vi "Decode.vi"(8 "error in (no error)":errorcluster, 11 "JSON in":string) -> (0 "error out":errorcluster, 3 "Variant out":variant)   [LabVIEW 2019, in "JSON.lvlib"]
doc: "Decodes the JSON string to a LabVIEW Variant where JSON objects are represented as LabVIEW Clusters.\n\nEmpty JSON objects (\"{}\") are represented as a Cluster with an U16 Enum <b>\"empty\"</b> placeholder. \nNull JSON values (\"NULL\") are represented as a U8 Enum <b>\"null\"</b> placeholder. \nElements in JSON arrays are represented as Variant values.\nTimestamps are JSON strings formatted as defined in RFC-3339 (\"yyyy-mm-ddThh:mm:ss.uuuuuu\").\n\nCreated by: Ryan Pacini"
uses:
  JSON.lvlib
  <vilib>/regexp/Match Regular Expression.xnode
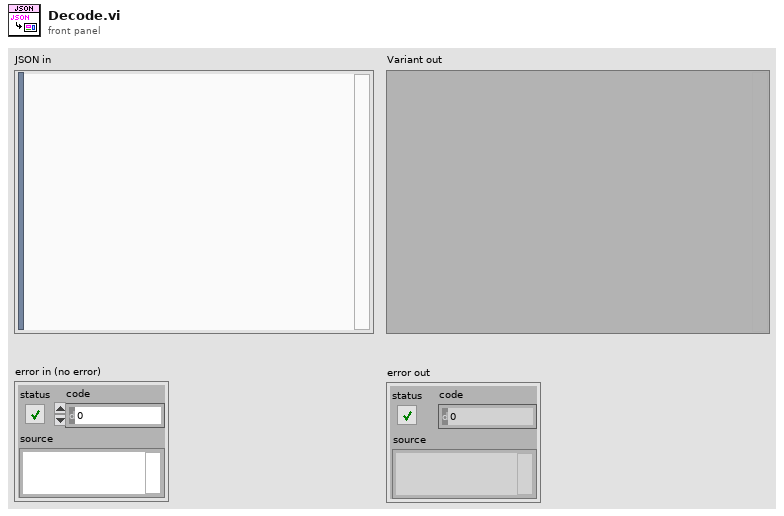
[diagram p1: front panel]
types:
  T1 = cluster{"k":string, "t":enum8{"root", "array", "object"}, "v":variant[]}[]
  T2 = cluster{"k":string, "t":enum8{"root", "array", "object"}, "v":variant[]}
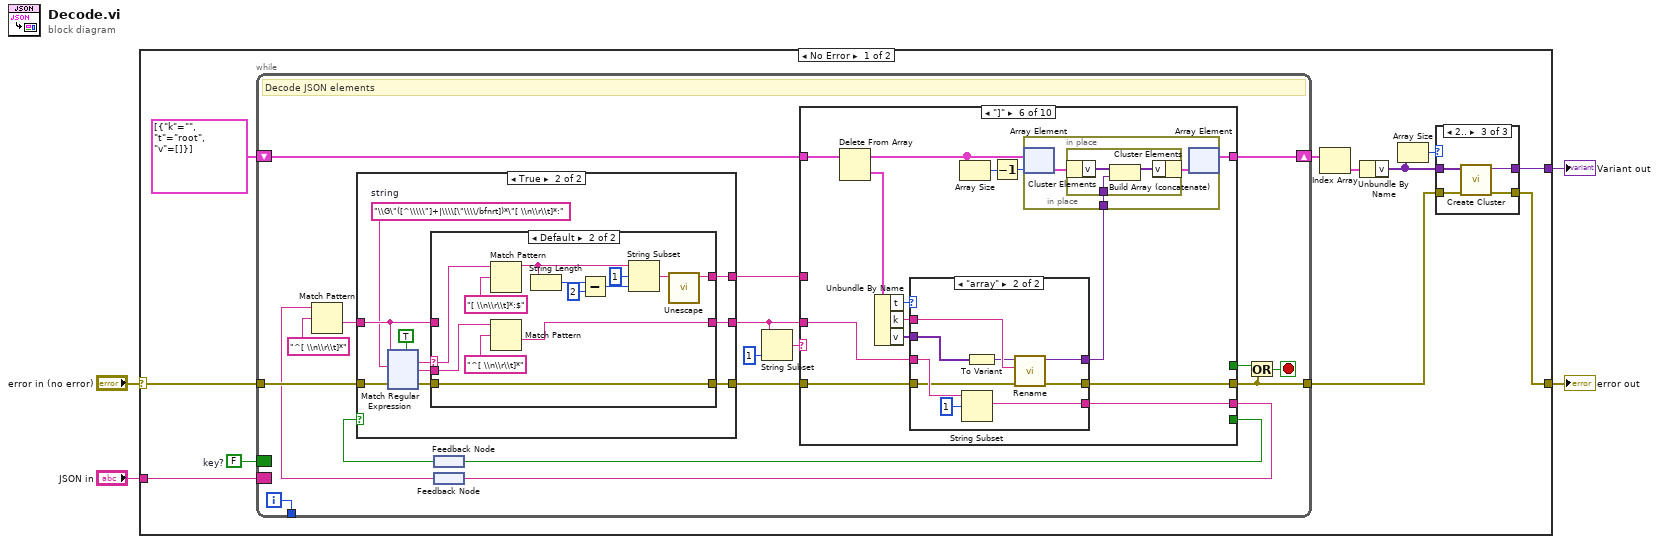
[diagram p0: block diagram]
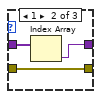
[diagram p3: hidden frame]
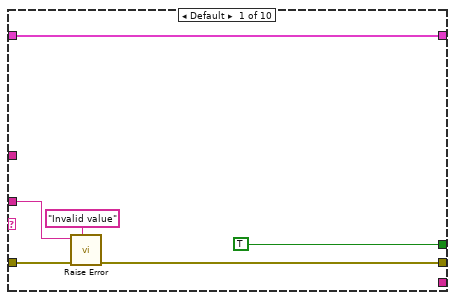
[diagram p4: hidden frame]
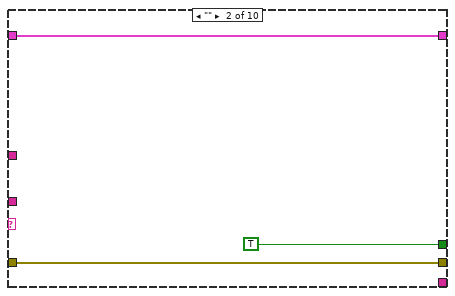
[diagram p5: hidden frame]
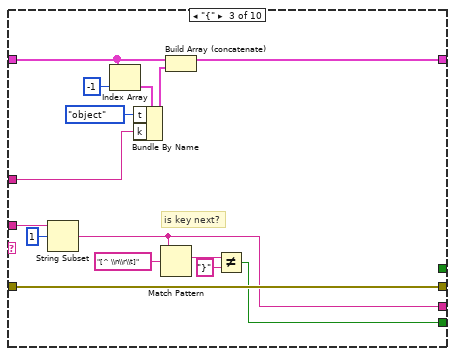
[diagram p6: hidden frame]
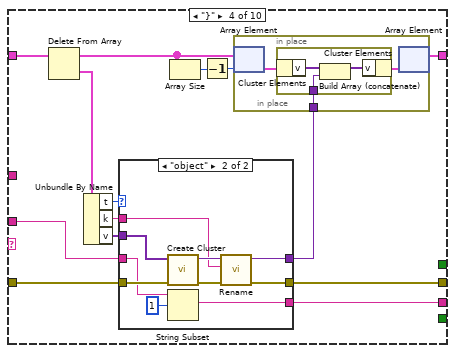
[diagram p7: hidden frame]
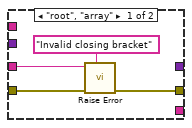
[diagram p8: hidden frame]
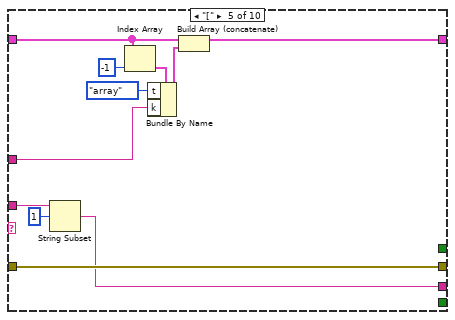
[diagram p9: hidden frame]
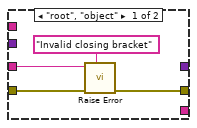
[diagram p10: hidden frame]
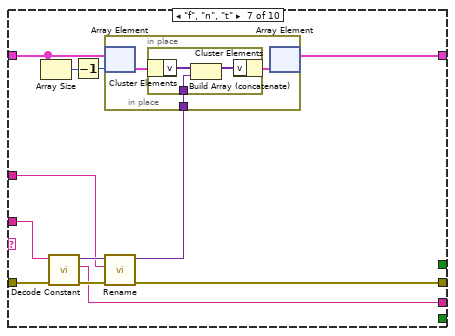
[diagram p11: hidden frame]
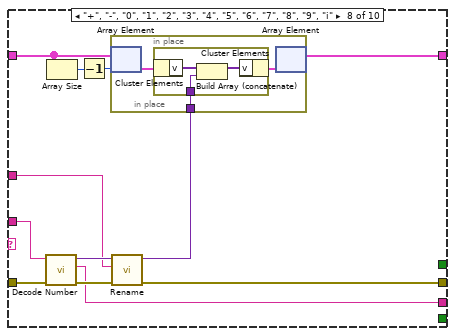
[diagram p12: hidden frame]
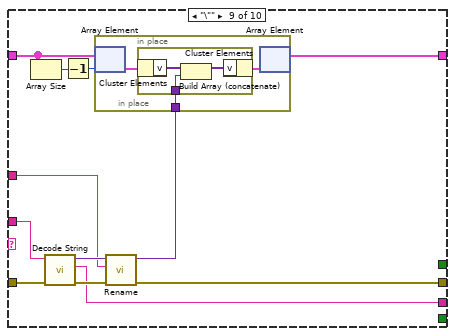
[diagram p13: hidden frame]
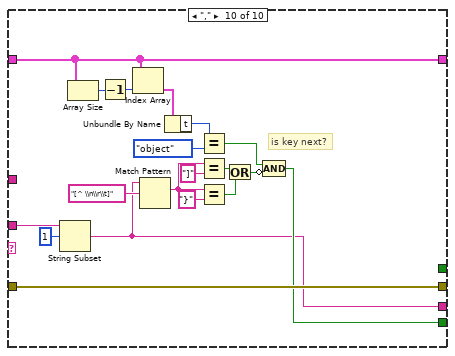
[diagram p14: hidden frame]
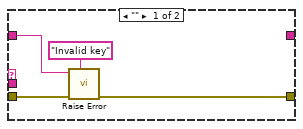
[diagram p16: hidden frame]
diagram:
  n1 = case shown="No Error" "error in (no error)" {
    selector: "error in (no error)" -> [w15 w360]
    tunnel: "JSON in" -> [w13 _]
    tunnel: [w5 w360] -> w2
    tunnel: [w8 _] -> w1
    frame No Error {
      w12 = FALSE  # key?
      n2 = while {
        tunnel: w15 -> [w41]
        shift-right: [w38] -> w11
        shift-left: T1 [{"k"="", "t"=enum."root", "v"=[]}] ("e") -> [w39]
        tunnel: [w36] -> w6
        border: w13 -> [_]
        border: w12 -> [_]
        tunnel: [w24] -> _
        i -> [w24]
        stop <- w34 stop-if-true
        # "Decode JSON elements"
        n3 = feedback #1() -> (w28:bool)
        n4 = feedback #2() -> (w32:string)
        n5 = Match Pattern(string=w32, regular expression="^[ \\n\\r\\t]*") -> (after substring=w31:string)  [unwired: 1 in, 3 out]
        n6 = case shown="True" w28 {
          tunnel: w41 -> [w218 w223]
          tunnel: w31 -> [w217 w225]
          tunnel: [w218 w226] -> w40
          tunnel: [_ w221] -> w37
          tunnel: [w217 w219] -> w27
          frame False {
          }
          frame True {
            w224 = "\\G\"([^\\\\\"]+|\\\\[\"\\\\/bfnrt])*\"[ \\n\\r\\t]*:"  # string
            n7 = xnode "Match Regular Expression"("input string"=w225, "regular expression"=w224, "error in"=w223, "multiline? (F)"=TRUE) -> ("whole match"=w227:string, "after match"=w220:string, "error out"=w222:errorcluster)  [unwired: 2 in, 2 out]
            n8 = case shown="Default" w227 {
              selector: w227 -> [_ w243]
              tunnel: w225 -> [w229 _]
              tunnel: [w231 w245] -> w226
              tunnel: w222 -> [w232 w245]
              tunnel: [_ w240] -> w221
              tunnel: w220 -> [_ w234]
              tunnel: [_ w233] -> w219
              frame "" {
                n9 = call "Raise Error.vi"("message"="Invalid key", "error in (no error)"=w232, "json"=w229) -> ("error out"=w231:errorcluster)  [unwired: 8 in]
              }
              frame Default {
                n10 = Match Pattern(string=w243, regular expression="[ \\n\\r\\t]*:$") -> (before substring=w239:string)  [unwired: 1 in, 3 out]
                n11 = Match Pattern(string=w234, regular expression="^[ \\n\\r\\t]*") -> (after substring=w233:string)  [unwired: 1 in, 3 out]
                n12 = String Length(string=w239) -> (length=w237:i32)
                n13 = Subtract(x=w237, y=2 ("x")) -> (x-y=w236:i32)
                n14 = String Subset(string=w239, offset (0)=1, length (rest)=w236) -> (substring=w241:string)
                n15 = call "Unescape.vi"("escaped string"=w241) -> ("string out"=w240:string)  [unwired: 9 in, 1 out]
              }
            }
          }
        }
        n16 = String Subset(string=w27, length (rest)=1 ("length (rest)")) -> (substring=w29:string)  [unwired: 1 in]
        n17 = case shown="\"]\"" w29 {
          tunnel: w40 -> [w44 w48 w65 w73 w110 w118 w155 w173 w191 w216]
          tunnel: [w43 w48 w65 w71 w110 w116 w148 w166 w184 w216] -> w36
          tunnel: w39 -> [w47 w50 w57 w79 w106 w124 w152 w169 w187 w206]
          tunnel: [w47 w50 w64 w74 w109 w119 w153 w168 w186 w206] -> w38
          tunnel: w37 -> [_ _ w60 _ w107 _ w146 w163 w181 _]
          tunnel: [_ _ w61 _ _ _ _ _ _ w207] -> w26
          tunnel: w27 -> [w42 _ w53 w68 w102 w112 w154 w172 w190 w201]
          tunnel: [TRUE TRUE _ _ _ _ _ _ _ _] -> w35
          tunnel: [_ _ w52 w67 w101 w111 w144 w164 w182 w199] -> w25
          frame Default {
            n18 = call "Raise Error.vi"("message"="Invalid value" ("source"), "error in (no error)"=w44, "json"=w42) -> ("error out"=w43:errorcluster)  [unwired: 8 in]
          }
          frame "" {
          }
          frame "{" {
            # "is key next?"
            n19 = String Subset(string=w53, offset (0)=1) -> (substring=w52:string)  [unwired: 1 in]
            n20 = Index Array(array=w57, index=-1) -> (element=w55:T2)
            n21 = Bundle By Name(cluster=w55, "t"=enum8{"root", "array", "object"}."object", "k"=w60) -> (w63:T2)
            n22 = Match Pattern(string=w52, regular expression="[^ \\n\\r\\t]") -> (match substring=w58:string)  [unwired: 1 in, 3 out]
            n23 = Build Array (concatenate)(w57, w63) -> (w64:T1)
            n24 = Not Equal?(x=w58, y="}") -> (x != y?=w61:bool)
          }
          frame "}" {
            n25 = Delete From Array(array=w79) -> (deleted portion=w78:T2, array with subset deleted=w75:T1)  [unwired: 2 in]
            n26 = Unbundle By Name(w78) -> ("t"=w69:enum8{"root", "array", "object"}, "k"=w70:string, "v"=w72:variant[])
            n27 = case shown="\"object\"" w69 {
              tunnel: w73 -> [w82 w93]
              tunnel: w72 -> [_ w84]
              tunnel: [w81 w91] -> w71
              tunnel: w70 -> [_ w89]
              tunnel: [_ w88] -> w66
              tunnel: w68 -> [w80 w85]
              tunnel: [_ w86] -> w67
              frame "root", "array" {
                n28 = call "Raise Error.vi"("message"="Invalid closing bracket", "error in (no error)"=w82, "json"=w80) -> ("error out"=w81:errorcluster)  [unwired: 8 in]
              }
              frame "object" {
                n29 = call "Create Cluster.vi"("error in (no error)"=w93, "elements"=w84) -> ("error out"=w92:errorcluster, "cluster"=w90:variant)  [unwired: 8 in]
                n30 = String Subset(string=w85, offset (0)=1) -> (substring=w86:string)  [unwired: 1 in]
                n31 = call "Rename.vi"("error in (no error)"=w92, "name"=w89, "variant in"=w90) -> ("error out"=w91:errorcluster, "variant out"=w88:variant)  [unwired: 7 in]
              }
            }
            n32 = Array Size(array=w75) -> (size(s)=w77:i32)
            n33 = Decrement(x=w77) -> (x-1=w76:i32)
            n34 = in-place {
              in-place-border: w66 -> [w95]
              n35 = in-place-array #3(w75, w76) -> (w96:T2)
              n36 = in-place {
                in-place-border: w95 -> [w97]
                n37 = in-place-cluster #4(w96) -> ("v"=w99:variant[])
                n38 = Build Array (concatenate)(w99, w97) -> (w98:variant[])
                n39 = in-place-cluster #4("v"=w98) -> (w94:T2)
              }
              n40 = in-place-array #3(w94) -> (w74:T1)  [unwired: 1 out]
            }
          }
          frame "[" {
            n41 = String Subset(string=w102, offset (0)=1) -> (substring=w101:string)  [unwired: 1 in]
            n42 = Index Array(array=w106, index=-1) -> (element=w105:T2)
            n43 = Bundle By Name(cluster=w105, "t"=enum8{"root", "array", "object"}."array", "k"=w107) -> (w108:T2)
            n44 = Build Array (concatenate)(w106, w108) -> (w109:T1)
          }
          frame "]" {
            n45 = Delete From Array(array=w124) -> (deleted portion=w123:T2, array with subset deleted=w120:T1)  [unwired: 2 in]
            n46 = Unbundle By Name(w123) -> ("t"=w113:enum8{"root", "array", "object"}, "k"=w115:string, "v"=w117:variant[])
            n47 = case shown="\"array\"" w113 {
              tunnel: w118 -> [w127 w129]
              tunnel: w117 -> [_ w131]
              tunnel: [w126 w137] -> w116
              tunnel: w115 -> [_ w136]
              tunnel: [_ w135] -> w114
              tunnel: w112 -> [w125 w133]
              tunnel: [_ w132] -> w111
              frame "root", "object" {
                n48 = call "Raise Error.vi"("message"="Invalid closing bracket", "error in (no error)"=w127, "json"=w125) -> ("error out"=w126:errorcluster)  [unwired: 8 in]
              }
              frame "array" {
                n49 = String Subset(string=w133, offset (0)=1) -> (substring=w132:string)  [unwired: 1 in]
                n50 = To Variant(anything=w131) -> (Variant=w130:variant)
                n51 = call "Rename.vi"("error in (no error)"=w129, "name"=w136, "variant in"=w130) -> ("error out"=w137:errorcluster, "variant out"=w135:variant)  [unwired: 7 in]
              }
            }
            n52 = Array Size(array=w120) -> (size(s)=w122:i32)
            n53 = Decrement(x=w122) -> (x-1=w121:i32)
            n54 = in-place {
              in-place-border: w114 -> [w139]
              n55 = in-place-array #5(w120, w121) -> (w140:T2)
              n56 = in-place {
                in-place-border: w139 -> [w141]
                n57 = in-place-cluster #6(w140) -> ("v"=w143:variant[])
                n58 = Build Array (concatenate)(w143, w141) -> (w142:variant[])
                n59 = in-place-cluster #6("v"=w142) -> (w138:T2)
              }
              n60 = in-place-array #5(w138) -> (w119:T1)  [unwired: 1 out]
            }
          }
          frame "f", "n", "t" {
            n61 = Array Size(array=w152) -> (size(s)=w151:i32)
            n62 = call "Decode Constant.vi"("error in (no error)"=w155, "JSON"=w154) -> ("error out"=w149:errorcluster, "Remaining JSON"=w144:string, "Value"=w147:variant)  [unwired: 7 in]
            n63 = Decrement(x=w151) -> (x-1=w150:i32)
            n64 = call "Rename.vi"("error in (no error)"=w149, "name"=w146, "variant in"=w147) -> ("error out"=w148:errorcluster, "variant out"=w145:variant)  [unwired: 7 in]
            n65 = in-place {
              in-place-border: w145 -> [w157]
              n66 = in-place-array #7(w152, w150) -> (w158:T2)
              n67 = in-place {
                in-place-border: w157 -> [w159]
                n68 = in-place-cluster #8(w158) -> ("v"=w161:variant[])
                n69 = Build Array (concatenate)(w161, w159) -> (w160:variant[])
                n70 = in-place-cluster #8("v"=w160) -> (w156:T2)
              }
              n71 = in-place-array #7(w156) -> (w153:T1)  [unwired: 1 out]
            }
          }
          frame "+", "-", "0", "1", "2", "3", "4", "5", "6", "7", "8", "9", "i" {
            n72 = call "Decode Number.vi"("error in (no error)"=w173, "json"=w172) -> ("error out"=w167:errorcluster, "remaining json"=w164:string, "value"=w165:variant)  [unwired: 7 in]
            n73 = Array Size(array=w169) -> (size(s)=w171:i32)
            n74 = Decrement(x=w171) -> (x-1=w170:i32)
            n75 = call "Rename.vi"("error in (no error)"=w167, "name"=w163, "variant in"=w165) -> ("error out"=w166:errorcluster, "variant out"=w162:variant)  [unwired: 7 in]
            n76 = in-place {
              in-place-border: w162 -> [w175]
              n77 = in-place-array #9(w169, w170) -> (w176:T2)
              n78 = in-place {
                in-place-border: w175 -> [w177]
                n79 = in-place-cluster #10(w176) -> ("v"=w179:variant[])
                n80 = Build Array (concatenate)(w179, w177) -> (w178:variant[])
                n81 = in-place-cluster #10("v"=w178) -> (w174:T2)
              }
              n82 = in-place-array #9(w174) -> (w168:T1)  [unwired: 1 out]
            }
          }
          frame "\"" {
            n83 = Array Size(array=w187) -> (size(s)=w189:i32)
            n84 = call "Decode String.vi"("error in (no error)"=w191, "json"=w190) -> ("error out"=w185:errorcluster, "remaining json"=w182:string, "value"=w183:variant)  [unwired: 7 in]
            n85 = Decrement(x=w189) -> (x-1=w188:i32)
            n86 = call "Rename.vi"("error in (no error)"=w185, "name"=w181, "variant in"=w183) -> ("error out"=w184:errorcluster, "variant out"=w180:variant)  [unwired: 7 in]
            n87 = in-place {
              in-place-border: w180 -> [w193]
              n88 = in-place-array #11(w187, w188) -> (w194:T2)
              n89 = in-place {
                in-place-border: w193 -> [w195]
                n90 = in-place-cluster #12(w194) -> ("v"=w197:variant[])
                n91 = Build Array (concatenate)(w197, w195) -> (w196:variant[])
                n92 = in-place-cluster #12("v"=w196) -> (w192:T2)
              }
              n93 = in-place-array #11(w192) -> (w186:T1)  [unwired: 1 out]
            }
          }
          frame "," {
            # "is key next?"
            n94 = String Subset(string=w201, offset (0)=1) -> (substring=w199:string)  [unwired: 1 in]
            n95 = Array Size(array=w206) -> (size(s)=w205:i32)
            n96 = Decrement(x=w205) -> (x-1=w204:i32)
            n97 = Index Array(array=w206, index=w204) -> (element=w215:T2)
            n98 = Match Pattern(string=w199, regular expression="[^ \\n\\r\\t]") -> (match substring=w202:string)  [unwired: 1 in, 3 out]
            n99 = Unbundle By Name(w215) -> ("t"=w214:enum8{"root", "array", "object"})
            n100 = Equal?(x=w214, y=enum8{"root", "array", "object"}."object") -> (x = y?=w209:bool)
            n101 = Equal?(x=w202, y="]") -> (x = y?=w211:bool)
            n102 = Equal?(x=w202, y="}") -> (x = y?=w210:bool)
            n103 = Or(x=w211, y=w210) -> (x .or. y?=w208:bool)
            n104 = Compound Arithmetic op=AND(w209, invert w208) -> (w207:bool)
          }
        }
        n105 = feedback-in #1(w26) -> ()
        n106 = feedback-in #2(w25) -> ()
        n107 = Or(x=w35, y=w36) -> (x .or. y?=w34:bool)
      }
      n108 = Index Array(array=w11) -> (element=w10:T2)  [unwired: 1 in]
      n109 = Unbundle By Name(w10) -> ("v"=w9:variant[])
      n110 = Array Size(array=w9) -> (size(s)=w7:i32)
      n111 = case shown="2.." w7 {
        tunnel: w9 -> [_ w19 w23]
        tunnel: [_ w18 w22] -> w8
        tunnel: w6 -> [w16 w17 w21]
        tunnel: [w16 w17 w20] -> w5
        frame ..0 {
        }
        frame 1 {
          n112 = Index Array(array=w19) -> (element=w18:variant)  [unwired: 1 in]
        }
        frame 2.. {
          n113 = call "Create Cluster.vi"("error in (no error)"=w21, "elements"=w23) -> ("error out"=w20:errorcluster, "cluster"=w22:variant)  [unwired: 8 in]
        }
      }
    }
    frame Error {
    }
  }
  "error out" <- w2
  "Variant out" <- w1
